vi "Message Window 2.vi"(8 "error in (no error)":errorcluster, 11 "Message string":string) -> (0 "error out (no error)":errorcluster, 3 "Ok ?":bool)   [LabVIEW 2020]
doc: "Use this template to create a dialog box with event handling."
uses:
  <vilib>/Utility/miscctls.llb/LVPointTypeDef.ctl
  Global Variables/General Globals.vi
panel:
  in  "Cancel":bool
  out "Message":string
  in  "OK":bool
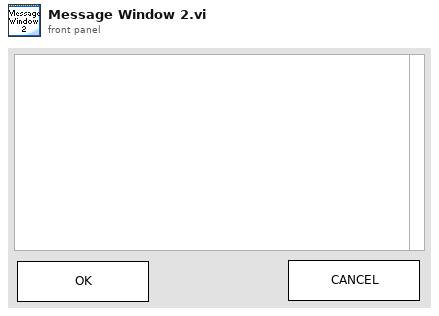
[diagram p1: front panel]
types:
  T1 = typedef "LVPointTypeDef.ctl" = cluster{"Horizontal":i16, "Vertical":i16}
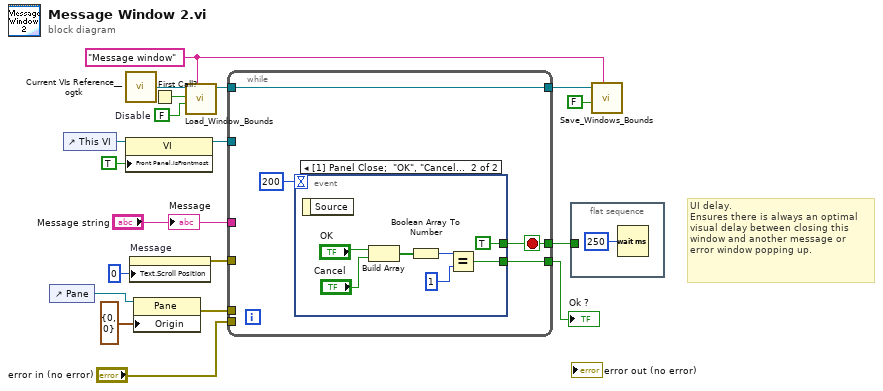
[diagram p0: block diagram]
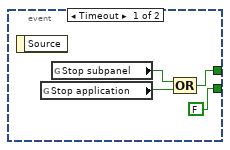
[diagram p2: hidden frame]
diagram:
  w7 = FALSE  # Disable
  w6 = "Message window" ("Window Name (i.e. Key)")
  # "UI delay.\nEnsures there is always an optimal visual delay between closing this window and another message or error window popping up."
  n1 = control-ref of="Pane"() -> (w11:refnum<vi>)
  n2 = control-ref of="This VI"() -> (w15:refnum<vi>)
  n3 = call <userlib>:"Current VIs Reference__ogtk.vi"() -> ("Current VI's reference"=w9:refnum<vi>)  [unwired: 5 in]
  n4 = property on="Property Node" class="VI"(reference=w15, "Front Panel.IsFrontmost"=TRUE ("Front Panel Window:Is Frontmost")) -> (reference out=w14:refnum<vi>)  [unwired: 1 in, 1 out]
  n5 = property on="Message" class="Str"("Text.Scroll Position"=u32 0) -> (error out=w17:errorcluster)  [unwired: 2 in, 1 out]
  n6 = property class="Pane"(reference=w11, "Origin"=T1 {"Horizontal"=0, "Vertical"=0}) -> (error out=w12:errorcluster)  [unwired: 1 in, 1 out]
  n7 = First Call?() -> (First Call?: T/F=w8:bool)
  n8 = call "Load_Window_Bounds.vi"("Window Name (i.e. Key)"=w6, "Disable"=w7, "First Call"=w8, "Window VI's Ref"=w9) -> ("reference out"=w4:refnum<vi>)  [unwired: 4 in, 3 out]
  n9 = while {
    tunnel: "Message string" -> [_]
    tunnel: w17 -> [_]
    tunnel: w12 -> [_]
    tunnel: w14 -> [_]
    tunnel: [w22] -> w10
    tunnel: w4 -> [w21]
    tunnel: [w21] -> w3
    tunnel: "error in (no error)" -> [_]
    tunnel: [w20] -> w1
    stop <- w22 stop-if-true
    n10 = event shown="[1] Panel Close;  \"OK\", \"Cancel\": Value Change" {
      selector: _ -> [_ _]
      dyn-events: _ -> [_ _]
      timeout: 200 -> [_ _]
      tunnel: [w25 TRUE ("Stop?")] -> w22
      tunnel: [FALSE w28] -> w20
      event Timeout {
        n11 = event-data() -> ()  [unwired: 1 in, 1 out]
        n12 = global read "General Globals.vi" "Stop application"() -> (w27:bool)
        n13 = global read "General Globals.vi" "Stop subpanel"() -> (w26:bool)
        n14 = Compound Arithmetic op=OR(w26, w27) -> (w25:bool)
      }
      event Panel Close; "OK", "Cancel": Value Change {
        n15 = event-data() -> ()  [unwired: 1 in, 1 out]
        n16 = Build Array("OK", "Cancel") -> (w31:bool[])
        n17 = Boolean Array To Number(Boolean array=w31) -> (number=w30:u32)
        n18 = Equal?(x=w30, y=u32 1) -> (x = y?=w28:bool)
      }
    }
  }
  "Ok ?" <- w1
  n19 = flat-sequence {
    tunnel: w10 -> [_]
    frame #0 {
      n20 = Wait (ms)(milliseconds to wait=u32 250) -> ()  [unwired: 1 out]
    }
  }
  n21 = call "Save_Windows_Bounds.vi"("Window Name (i.e. Key)"=w6, "Front Panel Window:Open"=FALSE, "Window VI's Ref"=w3) -> ()  [unwired: 8 in, 1 out]
  "Message" <- "Message string"
